vi "commandExit.vi"(8 "error in (no error)":errorcluster, 10 "CommandExit in":T1, 11 "M1M3SAL in":refnum<class "M1M3SAL.lvclass">) -> (0 "error out":errorcluster, 2 "CommandExit out":T1, 3 "M1M3SAL out":refnum<class "M1M3SAL.lvclass">)   [LabVIEW 2016, in "M1M3SupportCommunicator.lvlib" / "M1M3SAL.lvclass"]
uses:
  M1M3SAL.lvclass
  DataTypes/Topics/CommandExit.ctl
  DataTypes/Topics/Parts/CommandId.ctl
  DataTypes/MessageHeader.ctl
  DataTypes/MessageTypes.ctl
  DataTypes/MessageTopics.ctl
  Common_RT_Utilities/U8ArrayBuilderAutoIndexing/U8ArrayBuilderAutoIndexing.lvclass
  M1M3SupportCommunicator.lvlib
  DataTypes/Topics/M1M3SupportTopics.lvlib
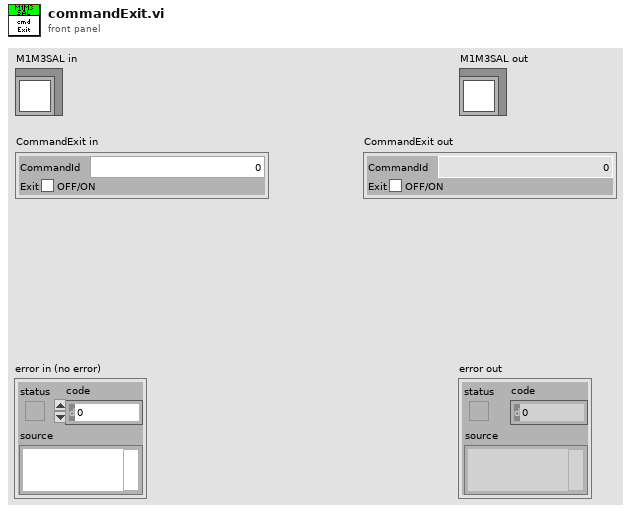
[diagram p1: front panel]
types:
  T1 = typedef "M1M3SupportTopics.lvlib/CommandExit.ctl" = cluster{"CommandId":T2, "Exit":bool}
  T2 = typedef "M1M3SupportTopics.lvlib/CommandId.ctl" = i32
  T3 = typedef "M1M3SupportCommunicator.lvlib/MessageHeader.ctl" = cluster{"Type":T4, "Topic":T5, "Size":i32}
  T4 = typedef "M1M3SupportCommunicator.lvlib/MessageTypes.ctl" = enum8{"None", "PutSample", "GetNextSample", "LogEvent", "GetEvent", "IssueCommand", "CommandId", "WaitForCompletion", "AcceptCommand", "AckCommand"}
  T5 = typedef "M1M3SupportCommunicator.lvlib/MessageTopics.ctl" = enum8{"None", "ForceActuatorData", "MirrorForceData", "HardpointData", "AirData", "DynamicData", "FPGAData", "IMSData", "ForceActuatorStatus", "ElevationData", "HardpointStatus", "HardpointActuatorChase", "AirStatus", "ForceActuatorSafetyChecks", "ForceActuatorTest", "ActuatorBroadcastCounter", "StatusChecks", "CellChecks", "HardpointActuatorBreakaway", "RaiseMirrorComplete", "ILCCommunication", "ElevationAngleChecks", "DetailedState", "ServoLoops", "ForceActuatorInfo", "LowerMirrorComplete", "HardpointActuatorInfo", "SettingsApplied", "ErrorCode", "StartupChecks", "SummaryState", "SettingVersions", "ActuatorTestStatus", "AppliedSettingsMatchStart", "Enable", "EnterMaintenance", "Standby", "AbortLowerM1M3", "ApplyAberrationByForces", "ApplyAOSCorrectionByBendingModes", "ClearAOSCorrection", "Start", "RaiseM1M3", "TestForceActuator", "LowerM1M3", "ApplyAOSCorrectionByForces", "Disable", "ApplyAberationByBendingMode", "TestHardpoint", "ManipulateM1M3", "ClearAberration", "Exit", "TestAir", "AbortRaiseM1M3", "MoveHardpointActuators", "ExitMaintenance", "Shutdown"}
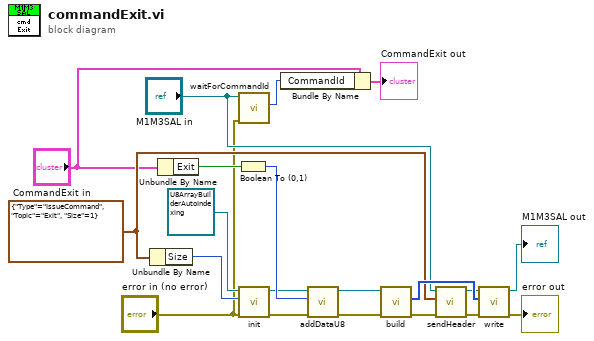
[diagram p0: block diagram]
diagram:
  w9 = T3 {"Type"=enum."IssueCommand", "Topic"=enum."Exit", "Size"=1} ("MessageHeader")
  n1 = Unbundle By Name(w9) -> ("Size"=w8:i32)
  n2 = Unbundle By Name("CommandExit in") -> ("Exit"=w16:bool)
  n3 = Boolean To (0,1)(Boolean=w16) -> (0, 1=w15:i16)
  n4 = call "waitForCommandId.vi"("error in (no error)"="error in (no error)", "M1M3SAL in"="M1M3SAL in") -> ("CommandId"=w5:T2)  [unwired: 7 in, 2 out]
  n5 = call "init.vi"("error in (no error)"="error in (no error)", "Size"=w8, "U8ArrayBuilderAutoIndexing in"=refnum<class "U8ArrayBuilderAutoIndexing.lvclass"> refnum ("RTUtilities.lvlib:U8ArrayBuilderAutoIndexing.lvclass")) -> ("error out"=w17:errorcluster, "U8ArrayBuilderAutoIndexing out"=w13:refnum<class "U8ArrayBuilderAutoIndexing.lvclass">)  [unwired: 7 in]
  n6 = Bundle By Name(cluster="CommandExit in", "CommandId"=w5) -> (→"CommandExit out":T1)
  n7 = call "addDataU8.vi"("error in (no error)"=w17, "Data"=w15, "U8ArrayBuilderAutoIndexing in"=w13) -> ("error out"=w18:errorcluster, "U8ArrayBuilderAutoIndexing out"=w12:refnum<class "U8ArrayBuilderAutoIndexing.lvclass">)  [unwired: 7 in]
  n8 = call "build.vi"("error in (no error)"=w18, "U8ArrayBuilderAutoIndexing in"=w12) -> ("error out"=w19:errorcluster, "Array"=w11:u8[])  [unwired: 7 in, 1 out]
  n9 = call "sendHeader.vi"("error in (no error)"=w19, "MessageHeader"=w9, "M1M3SAL in"="M1M3SAL in") -> ("error out"=w20:errorcluster, "M1M3SAL out"=w10:refnum<class "M1M3SAL.lvclass">)  [unwired: 7 in]
  n10 = call "write.vi"("error in (no error)"=w20, "Data"=w11, "M1M3SAL in"=w10) -> ("error out"=→"error out":errorcluster, "M1M3SAL out"=→"M1M3SAL out":refnum<class "M1M3SAL.lvclass">)  [unwired: 7 in]
